vi "Test Assert Array Not Contains.vi"(8 "error in (no error)":errorcluster) -> (0 "error out":errorcluster)   [LabVIEW 2013]
uses:
  classes/Assert/Assert.lvclass
  classes/Test/Test.lvclass
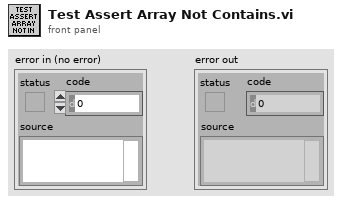
[diagram p1: front panel]
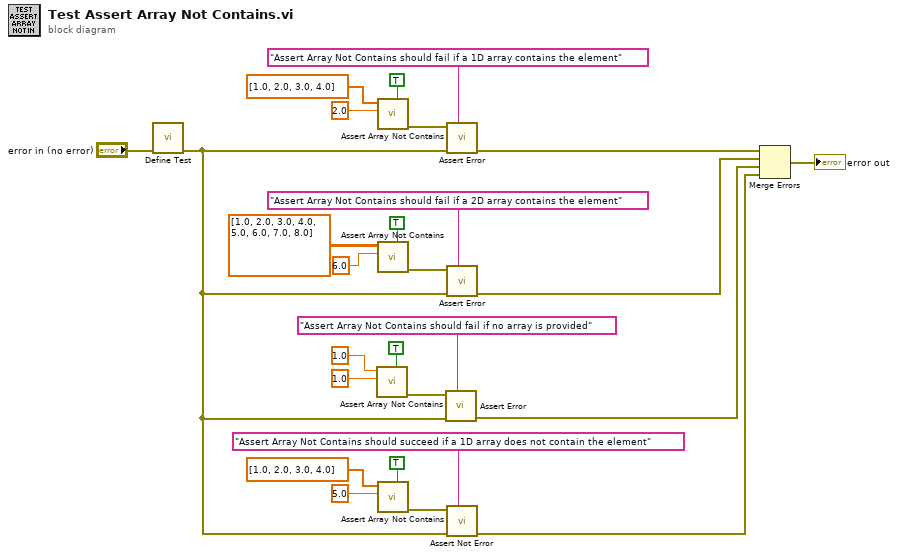
[diagram p0: block diagram]
diagram:
  n1 = call "Define Test.vi"("error in (no error)"="error in (no error)") -> ("error out"=w11:errorcluster)  [unwired: 9 in, 1 out]
  n2 = call "Assert Array Not Contains.vi"("Assert Only? (F)"=TRUE, "Element"=1.0 ("Count"), "Array"=1.0 ("element")) -> ("error out"=w15:errorcluster)  [unwired: 7 in, 1 out]
  n3 = call "Assert Array Not Contains.vi"("Assert Only? (F)"=TRUE, "Element"=2.0 ("element"), "Array"=dbl[] [1.0, 2.0, 3.0, 4.0] ("initialized array")) -> ("error out"=w27:errorcluster)  [unwired: 7 in, 1 out]
  n4 = call "Assert Array Not Contains.vi"("Assert Only? (F)"=TRUE, "Element"=6.0 ("Count"), "Array"=dbl[][] [[1.0, 2.0, 3.0, 4.0], [5.0, 6.0, 7.0, 8.0]] ("initialized array")) -> ("error out"=w19:errorcluster)  [unwired: 7 in, 1 out]
  n5 = call "Assert Array Not Contains.vi"("Assert Only? (F)"=TRUE, "Element"=5.0 ("element"), "Array"=dbl[] [1.0, 2.0, 3.0, 4.0] ("initialized array")) -> ("error out"=w1:errorcluster)  [unwired: 7 in, 1 out]
  n6 = call "Assert Error.vi"("Label"="Assert Array Not Contains should fail if no array is provided", "error in (no error)"=w11, "Error?"=w15) -> ("error out"=w13:errorcluster)  [unwired: 7 in, 1 out]
  n7 = call "Assert Error.vi"("Label"="Assert Array Not Contains should fail if a 1D array contains the element", "error in (no error)"=w11, "Error?"=w27) -> ("error out"=w23:errorcluster)  [unwired: 7 in, 1 out]
  n8 = call "Assert Error.vi"("Label"="Assert Array Not Contains should fail if a 2D array contains the element", "error in (no error)"=w11, "Error?"=w19) -> ("error out"=w18:errorcluster)  [unwired: 7 in, 1 out]
  n9 = call "Assert Not Error.vi"("Label"="Assert Array Not Contains should succeed if a 1D array does not contain the element", "error in (no error)"=w11, "Not Error?"=w1) -> ("error out"=w10:errorcluster)  [unwired: 7 in, 1 out]
  n10 = Merge Errors(w23, w18, w13, w10) -> (→"error out":errorcluster)
